vi "Get all Object Item Offsets.vi"(8 "error in (no error)":errorcluster, 10 "Offset":i32, 11 "JSON":string) -> (0 "error out":errorcluster, 1 "Items":T1[](array[typedef]), 2 "Offset past Object":i32)   [LabVIEW 2015, in "JSONtext.lvlib"]
uses:
  JSONtext.lvlib
  Found Items.ctl
  Parsing State.ctl
  Advance past Number.vi
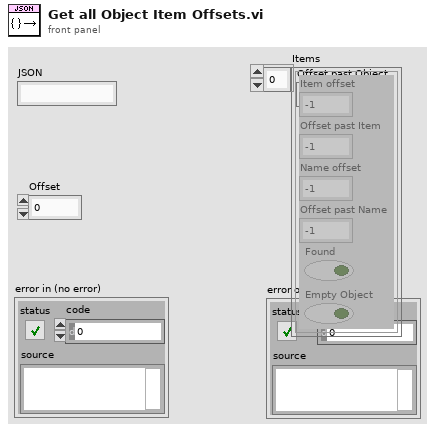
[diagram p1: front panel]
types:
  T1 = typedef "JSONtext.lvlib/Found Items.ctl" = cluster{"Item offset":i32, "Offset past Item":i32, "Name offset":i32, "Offset past Name":i32, "Found":bool, "Empty Object":bool}
  T2 = typedef "JSONtext.lvlib/Parsing State.ctl" = enum16{"Parser Error", "Object", "Array", "String", "Number/Other", "Leading Whitespace", "Object end", "Array end", "Value end"}
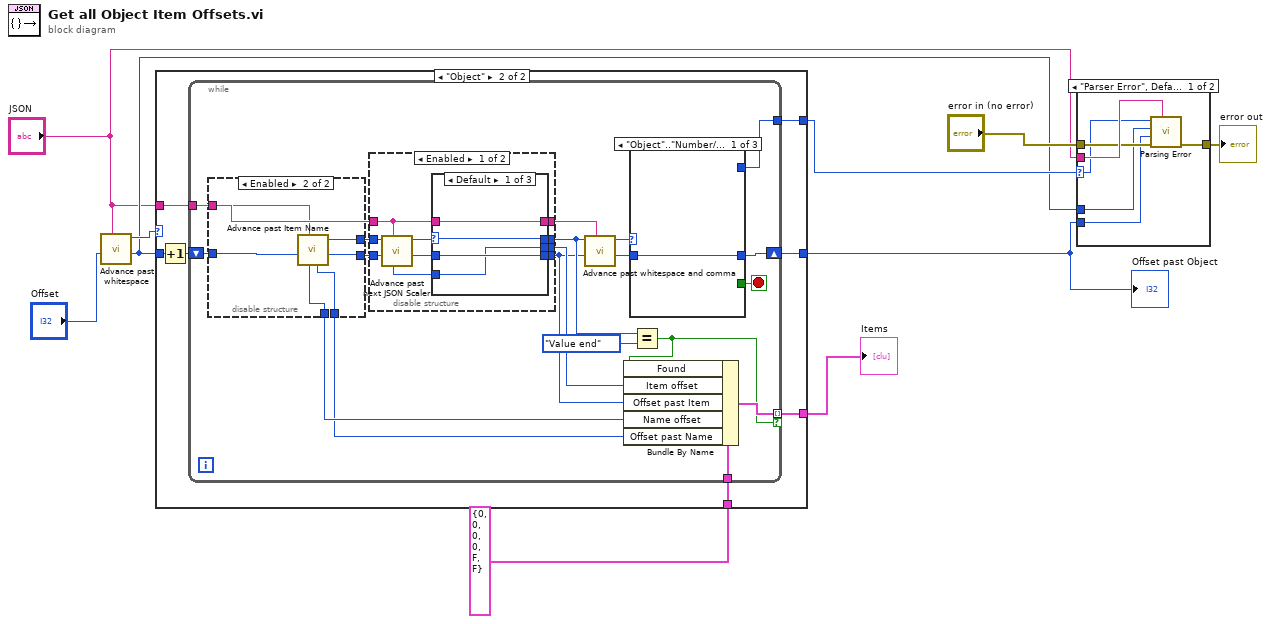
[diagram p0: block diagram]
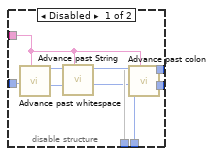
[diagram p4: hidden frame]
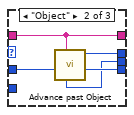
[diagram p5: hidden frame]
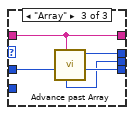
[diagram p6: hidden frame]
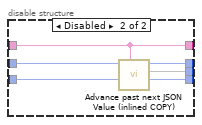
[diagram p7: hidden frame]
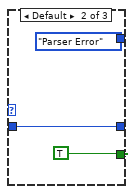
[diagram p8: hidden frame]
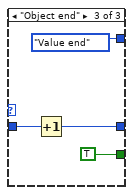
[diagram p9: hidden frame]
diagram:
  n1 = call "Advance past whitespace.vi"("JSON"="JSON", "Offset"="Offset") -> ("Offset of first non-whitespace"=w4:i32, "Parser State"=w9:T2)  [unwired: 8 in]
  n2 = case shown="\"Object\"" w9 {
    selector: w9 -> [w12 _]
    tunnel: [w12 w19] -> w5
    tunnel: w4 -> [w11 w17]
    tunnel: "JSON" -> [_ w16]
    tunnel: [w11 w15] -> w6
    tunnel: [_ w14] -> w2
    tunnel: T1 {"Item offset"=0, "Offset past Item"=0, "Name offset"=0, "Offset past Name"=0, "Found"=FALSE, "Empty Object"=FALSE} -> [_ w13]
    frame "Parser Error", Default {
    }
    frame "Object" {
      n3 = Increment(x=w17) -> (x+1=w18:i32)
      n4 = while {
        shift-right: [w36] -> w15
        shift-left: w18 -> [w33]
        tunnel: w16 -> [w29]
        tunnel: [w34] -> w19
        tunnel: [w24] -> w14 mode=indexing if=w23
        tunnel: w13 -> [w20]
        stop <- w35 stop-if-true
        n5 = disable-structure shown="Enabled" {
          disable-tunnel: w33 -> [w46 w51]
          disable-tunnel: [w43 w53] -> w31
          disable-tunnel: [w42 w52] -> w30
          disable-tunnel: w29 -> [w41 w50]
          disable-tunnel: [w40 w49] -> w22
          disable-tunnel: [w39 w48] -> w21
          frame Disabled {
            n6 = call "Advance past whitespace.vi"("JSON"=w41, "Offset"=w46) -> ("Offset of first non-whitespace"=w45:i32, "Parser State"=w44:T2)  [unwired: 8 in]
            n7 = call "Advance past String.vi"("JSON"=w41, "Offset"=w45, "State in"=w44) -> ("Offset past match"=w39:i32, 2:w40, "State"=w47:T2)  [unwired: 5 in, 1 out]
            n8 = call "Advance past colon.vi"("JSON"=w41, "Offset"=w39, "State"=w47) -> ("index"=w42:i32, "State"=w43:T2)  [unwired: 7 in]
          }
          frame Enabled {
            n9 = call "Advance past Item Name.vi"("JSON"=w50, "Offset"=w51) -> ("Offset past colon"=w52:i32, "State"=w53:T2, "Offset past Name"=w48:i32, "Name start out"=w49:i32)  [unwired: 6 in]
          }
        }
        n10 = disable-structure shown="Enabled" {
          disable-tunnel: [w63 w78] -> w32
          disable-tunnel: w31 -> [w61 w80]
          disable-tunnel: w30 -> [w60 w79]
          disable-tunnel: w29 -> [w58 w78]
          disable-tunnel: [w57 w81] -> w28
          disable-tunnel: [w56 w82] -> w26
          disable-tunnel: [w55 w83] -> w25
          frame Enabled {
            n11 = call "Advance past next JSON Scaler.vi"("JSON"=w58, "Offset"=w60, "Parser State in"=w61) -> ("index"=w59:i32, "Parser State"=w62:T2, "Value start"=w54:i32)  [unwired: 6 in]
            n12 = case shown="Default" w62 {
              selector: w62 -> [w66 _ _]
              tunnel: w59 -> [w65 w72 w77]
              tunnel: [w66 w71 w76] -> w57
              tunnel: [w65 w70 w75] -> w55
              tunnel: w58 -> [w67 w69 w74]
              tunnel: [w67 w69 w74] -> w63
              tunnel: [w64 w68 w73] -> w56
              tunnel: w54 -> [w64 _ _]
              frame Default {
              }
              frame "Object" {
                n13 = call "Advance past Object.vi"("JSON"=w69, "Offset"=w72) -> ("Offset past Object"=w70:i32, "State"=w71:T2, "Object Start"=w68:i32)  [unwired: 7 in]
              }
              frame "Array" {
                n14 = call "Advance past Array.vi"("JSON"=w74, "Offset"=w77) -> ("Offset past Array"=w75:i32, "State"=w76:T2, "Array Start"=w73:i32)  [unwired: 7 in]
              }
            }
          }
          frame Disabled {
            n15 = call "Advance past next JSON Value (inlined COPY).vi"("JSON"=w78, "Offset"=w79, "State"=w80) -> ("Offset"=w83:i32, 2:w82, "State"=w81:T2)  [unwired: 4 in, 2 out]
          }
        }
        n16 = call "Advance past whitespace and comma.vi"("JSON"=w32, "Offset"=w25, "State in"=w28) -> ("Offset past match"=w38:i32, "State"=w37:T2)  [unwired: 7 in]
        n17 = case shown="\"Object\"..\"Number/Other\"" w37 {
          tunnel: [_ TRUE TRUE] -> w35
          tunnel: [_ Parsing_State."Parser Error" Parsing_State."Value end"] -> w34
          tunnel: w38 -> [w84 w85 w89]
          tunnel: [w84 w85 w88] -> w36
          frame "Object".."Number/Other" {
          }
          frame Default {
          }
          frame "Object end" {
            n18 = Increment(x=w89) -> (x+1=w88:i32)
          }
        }
        n19 = Equal?(x=w28, y=Parsing_State."Value end") -> (x = y?=w23:bool)
        n20 = Bundle By Name(cluster=w20, "Found"=w23, "Item offset"=w26, "Offset past Item"=w25, "Name offset"=w22, "Offset past Name"=w21) -> (w24:T1)
      }
    }
  }
  "Offset past Object" <- w6
  "Items" <- w2
  n21 = case shown="\"Parser Error\", Default" w5 {
    selector: w5 -> [w92 _]
    tunnel: "JSON" -> [w97 _]
    tunnel: "error in (no error)" -> [w96 w98]
    tunnel: [w95 w98] -> w8
    tunnel: w4 -> [w94 _]
    tunnel: w6 -> [w93 _]
    frame "Parser Error", Default {
      n22 = call "Parsing Error.vi"("JSON"=w97, "error in (no error)"=w96, "Offset past match"=w93, "Value start"=w94, "State"=w92) -> ("error out"=w95:errorcluster)  [unwired: 6 in]
    }
    frame "Value end" {
    }
  }
  "error out" <- w8
